vi "Write AI Data.vi"(8 "error in (no error)":errorcluster, 10 "AI Data":dbl[](array[numeric]), 11 "DAQ Data in":refnum<class "DAQ Data.lvclass">) -> (0 "error out":errorcluster, 3 "DAQ Data out":refnum<class "DAQ Data.lvclass">)   [LabVIEW 2022 SP3, in "DAQ Data.lvclass"]
uses:
  DAQ Data.lvclass
  DAQ Data.lvclass/DAQ Data.ctl
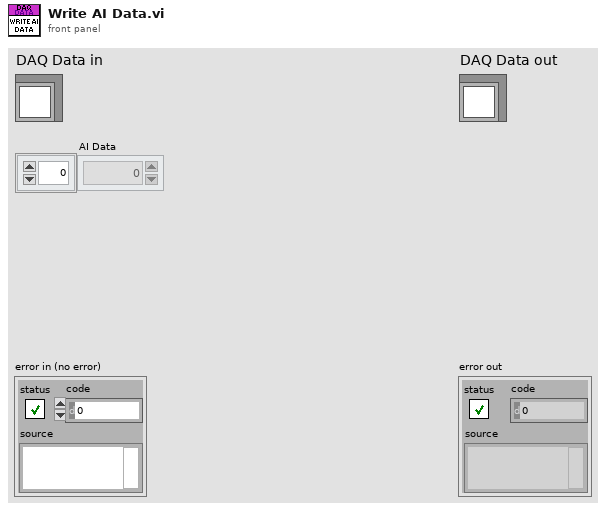
[diagram p1: front panel]
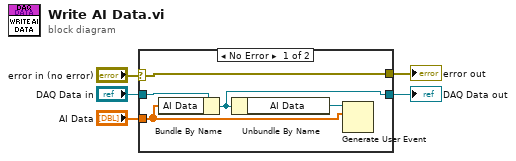
[diagram p0: block diagram]
diagram:
  n1 = case shown="No Error" "error in (no error)" {
    selector: "error in (no error)" -> [w10 w11]
    tunnel: [w10 w11] -> w4
    tunnel: [w7 w12] -> w2
    tunnel: "DAQ Data in" -> [w9 w12]
    tunnel: "AI Data" -> [w6 _]
    frame No Error {
      n2 = Bundle By Name(cluster=w9, "AI Data"=w6) -> (w7:refnum<class "DAQ Data.lvclass">)
      n3 = Unbundle By Name(w7) -> ("AI Data"=w8:refnum<user-event>)
      n4 = Generate User Event(user event=w8, event data cluster=w6) -> ()  [unwired: 2 in, 2 out]
    }
    frame Error {
    }
  }
  "error out" <- w4
  "DAQ Data out" <- w2
